vi "WPI_JoystickMecanumCartesianMapping.vi"(6 "Max Output":dbl=1.0, 7 "Gyro Angle":dbl, 8 "Rotation":dbl, 9 "Y":dbl, 10 "X":dbl) -> (0 "Rear Right":dbl, 1 "Rear Left":dbl, 2 "Front Right":dbl, 3 "Front Left":dbl)   [LabVIEW 2017]
doc: "Maps the joystick inputs for holonomic driving. Holonomic driving allows you to move the robot in any direction without first rotating or maneuvering the robot.\n\nThis VI assumes the robot to have either four omni-directional wheels and four motors mounted at 45 degree angles in the four corners of a square frame or to have four mecanum wheels driven by four motors."
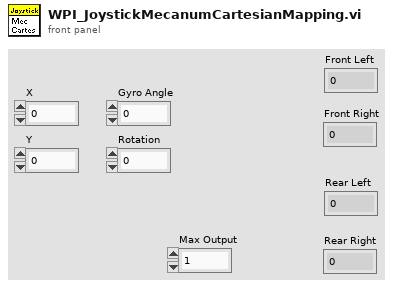
[diagram p1: front panel]
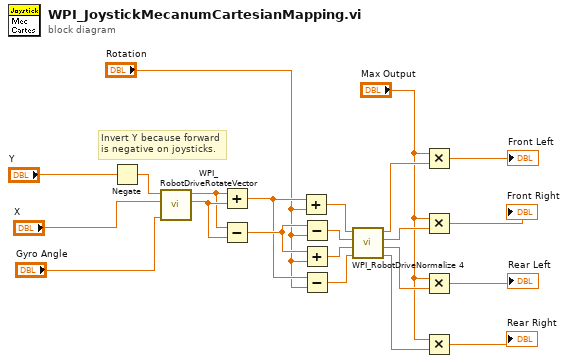
[diagram p0: block diagram]
diagram:
  # "Invert Y because forward is negative on joysticks."
  n1 = Negate(x="Y") -> (-x=w22:dbl)
  n2 = call <vilib>:"WPI_RobotDriveRotateVector.vi"("Angle"="Gyro Angle", "X"="X", "Y"=w22) -> ("X'"=w15:dbl, "Y'"=w14:dbl)  [unwired: 7 out]
  n3 = Add(x=w14, y=w15) -> (x+y=w17:dbl)
  n4 = Subtract(x=w14, y=w15) -> (x-y=w19:dbl)
  n5 = Add(x=w17, y="Rotation") -> (x+y=w21:dbl)
  n6 = Subtract(x=w19, y="Rotation") -> (x-y=w20:dbl)
  n7 = Add(x=w19, y="Rotation") -> (x+y=w18:dbl)
  n8 = Subtract(x=w17, y="Rotation") -> (x-y=w16:dbl)
  n9 = call <vilib>:"WPI_RobotDriveNormalize 4.vi"("D"=w16, "C"=w18, "B"=w20, "A"=w21) -> ("D'"=w10:dbl, "C'"=w11:dbl, "B'"=w12:dbl, "A'"=w13:dbl)
  n10 = Multiply(x="Max Output", y=w13) -> (x*y=→"Front Left":dbl)
  n11 = Multiply(x="Max Output", y=w12) -> (x*y=→"Front Right":dbl)
  n12 = Multiply(x="Max Output", y=w11) -> (x*y=→"Rear Left":dbl)
  n13 = Multiply(x="Max Output", y=w10) -> (x*y=→"Rear Right":dbl)
